vi "Final V1.vi"() -> ()   [LabVIEW 2021]
uses:
  <vilib>/MakerHub/LINX/Public/Sensors/Accelerometer/MPU60X0/AccelFullScaleRanges.ctl
  <vilib>/MakerHub/LINX/Public/Sensors/Accelerometer/MPU60X0/Clock Source.ctl
  <vilib>/MakerHub/LINX/Public/Sensors/Accelerometer/MPU60X0/DeviceAddresses.ctl
  <vilib>/MakerHub/LINX/Public/Sensors/Accelerometer/MPU60X0/GyroFullScaleRanges.ctl
  <vilib>/MakerHub/LINX/Public/Utilities/Open Serial.vi
  <vilib>/MakerHub/LINX/Public/Sensors/Motion/Servo/Servo Open One Channel.vi
  <vilib>/MakerHub/LINX/Public/Sensors/Motion/Servo/Servo Set Pulse Width One Channel.vi
  <vilib>/MakerHub/LINX/Public/Sensors/Motion/Servo/Servo Close One Channel.vi
  <vilib>/MakerHub/LINX/Public/Sensors/Motion/Servo/Servo.lvlib
  <vilib>/MakerHub/LINX/LMH-LINX.lvlib
  <vilib>/MakerHub/LINX/Public/Sensors/Accelerometer/MPU60X0/MPU60X0.lvlib
  <vilib>/Analysis/NI_AALPro.lvlib
panel:
  out "z position":dbl[](graph)
  out "y position":dbl[](graph)
  out "x position":dbl[](graph)
  out "acceleration graph":T1(graph)
  out "Acceleration Data (g)":T1
  in  "Servo 2":dbl(knob) scale=500.0..2400.0
  in  "Servo 1":dbl(knob) scale=500.0..2400.0
  in  "Stop Button":bool
  in  "Reset":bool
  in  "Serial Port":refnum<visa-resource-name>
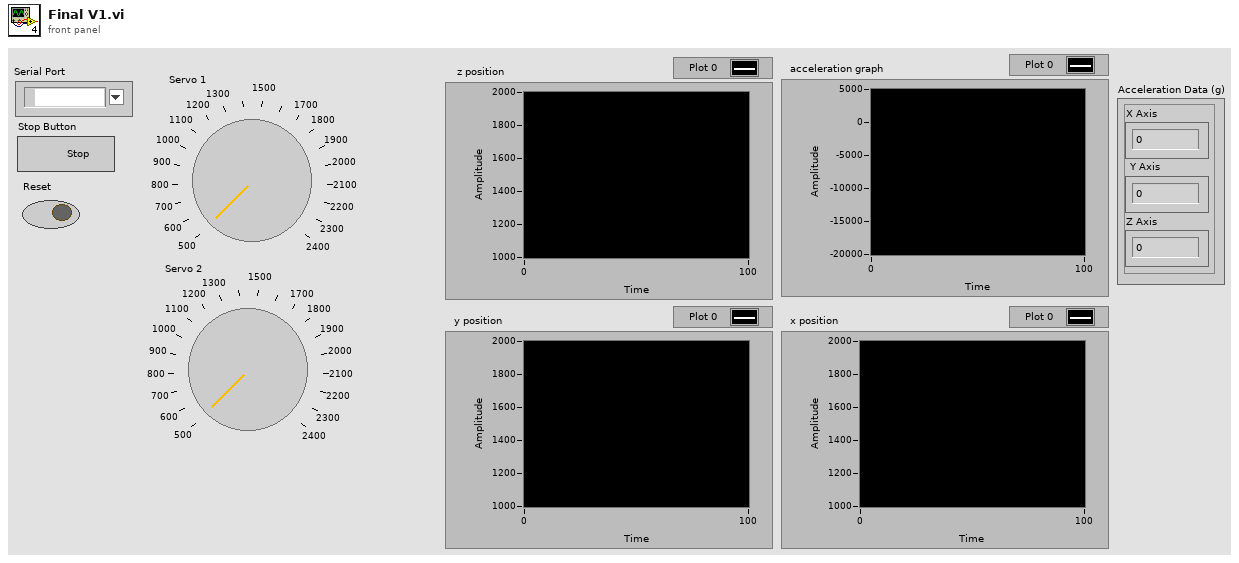
[diagram p1: front panel]
types:
  T1 = cluster{"X Axis":i16, "Y Axis":i16, "Z Axis":i16}
  T2 = typedef "LMH-LINX.lvlib/MPU60X0.lvlib/DeviceAddresses.ctl" = enum16{"0x68", "0x69"}
  T3 = typedef "LMH-LINX.lvlib/MPU60X0.lvlib/Clock Source.ctl" = enum8{"Internal 8MHz Osc", "PLL with X Gyro Ref", "PLL with Y Gyro Ref", "PLL with Z Gyro Ref", "PLL with ext 32.768 KHz Ref", "PLL with ext 19.2 MHz Ref", "Reserved", "Hold in reset"}
  T4 = typedef "LMH-LINX.lvlib/MPU60X0.lvlib/AccelFullScaleRanges.ctl" = enum16{"±2g", "±4g", "±8g", "±16g"}
  T5 = typedef "LMH-LINX.lvlib/MPU60X0.lvlib/GyroFullScaleRanges.ctl" = enum8{"±250 °/s", "±500 °/s", "±1000 °/s", "±2000 °/s"}
  T6 = typedef "LMH-LINX.lvlib/LINX Ref.ctl" = cluster{"IO":T7, "Interface":T8, "LINX Device Config":T9}
  T7 = typedef "LMH-LINX.lvlib/Platform.ctl" = enum16{"Remote", "Local"}
  T8 = typedef "LMH-LINX.lvlib/Interface.ctl" = enum16{"Serial", "TCP"}
  T9 = typedef "LMH-LINX.lvlib/Device.lvlib/LINX Device Config.ctl" = cluster{"Interface":T8, "COM Port":refnum<visa-resource-name>, "TCP Configuration":T10, "Device Family":u8, "Device ID":u8, "Device Name":string, "TCP Ref":refnum<k5>, "Channels":T11}
  T10 = typedef "LMH-LINX.lvlib/Device.lvlib/TCP Config.ctl" = cluster{"IP Address":string, "Port":u16}
  T11 = typedef "LMH-LINX.lvlib/Channels.ctl" = cluster{"DI":u8[], "DO":u8[], "AI":u8[], "AO":u8[], "PWM":u8[], "QE":u8[], "UART":u8[], "I2C 2":u8[], "SPI":u8[], "CAN":u8[], "Servo":u8[], "AI Ref (V)":dbl, "AI Resolution (Bits)":u8, "AO Ref (V)":dbl, "AO Resolution (Bits)":u8}
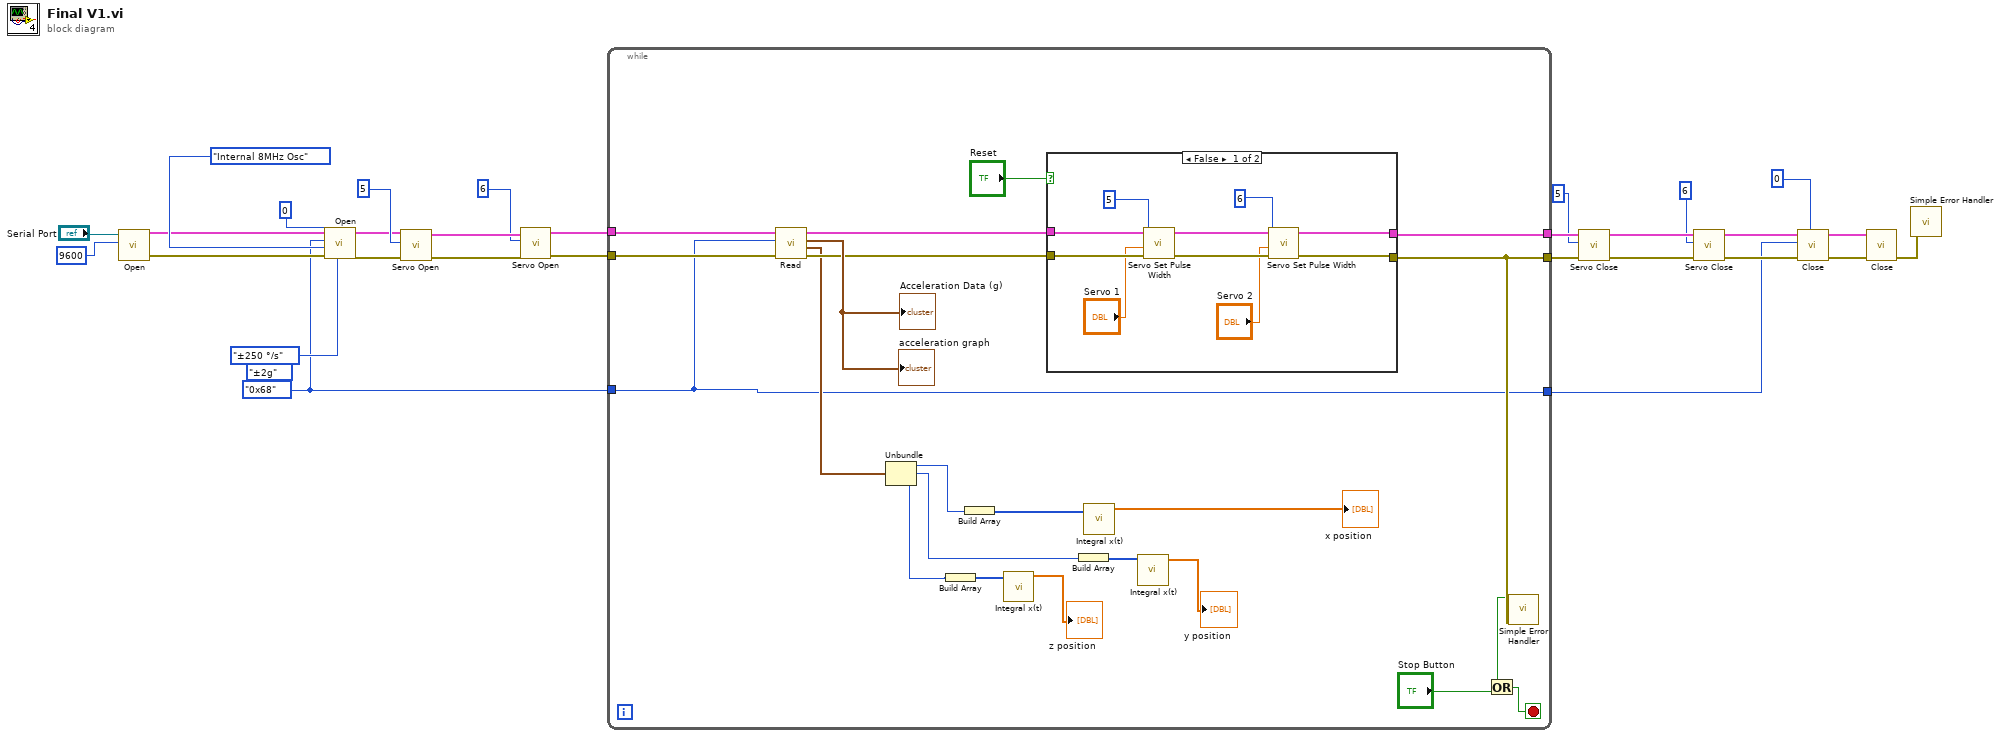
[diagram p0: block diagram]
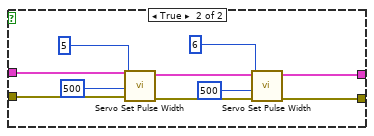
[diagram p2: hidden frame]
diagram:
  w7 = DeviceAddresses."0x68" ("I2C Slave Address")
  (unwired) GyroFullScaleRanges."±250 °/s" ("Gyro Full Scale Range")
  n1 = call-poly <vilib>:"Open.vi"("Baud Rate Override"=u32 9600, "Serial Port"="Serial Port") -> ("Error Out"=w8:errorcluster, "LINX Resource"=w11:T6)  [unwired: 7 in, 1 out]
  n2 = call <vilib>:"Open.vi"("Accel Full Scale Range"=AccelFullScaleRanges."±2g", "I2C Channel"=u8 0, "Error In"=w8, "Clock Source"=Clock_Source."Internal 8MHz Osc", "I2C Slave Address"=w7, "LINX Resource"=w11) -> ("Error Out"=w9:errorcluster, "LINX Resource"=w10:T6)  [unwired: 4 in]
  n3 = call-poly <vilib>:"Servo Open.vi"("Error In"=w9, "Servo Channel"=u8 5, "LINX Resource"=w10) -> ("Error Out"=w23:errorcluster, "LINX Resource"=w27:T6)  [unwired: 7 in]
  n4 = call-poly <vilib>:"Servo Open.vi"("Error In"=w23, "Servo Channel"=u8 6, "LINX Resource"=w27) -> ("Error Out"=w22:errorcluster, "LINX Resource"=w26:T6)  [unwired: 7 in]
  n5 = while {
    tunnel: w26 -> [w44]
    tunnel: [w50] -> w25
    tunnel: w22 -> [w42]
    tunnel: [w49] -> w21
    tunnel: w7 -> [w30]
    tunnel: [w30] -> w1
    stop <- w48 stop-if-true
    n6 = call <vilib>:"Read.vi"("Error In"=w42, "I2C Slave Address"=w30, "LINX Resource"=w44) -> ("Error Out"=w41:errorcluster, "Gyro  Data (dps)"=w34:T1, "Acceleration Data (g)"=→"Acceleration Data (g)" →"acceleration graph":T1, "LINX Resource"=w43:T6)  [unwired: 4 in, 1 out]
    n7 = Unbundle(w34) -> ("X Axis"=w40:i16, "Y Axis"=w33:i16, "Z Axis"=w35:i16)
    n8 = Build Array(w35) -> (w36:i16[])
    n9 = Build Array(w40) -> (w32:i16[])
    n10 = call <vilib>:"Integral x(t).vi"("X"=w36) -> ("Integral X"=→"z position":dbl[])  [unwired: 9 in, 1 out]
    n11 = case shown="False" "Reset" {
      tunnel: w43 -> [w59 w71]
      tunnel: [w58 w69] -> w50
      tunnel: w41 -> [w57 w68]
      tunnel: [w56 w66] -> w49
      frame False {
        n12 = call-poly <vilib>:"Servo Set Pulse Width.vi"("Error In"=w57, "Pulse Width (uS)"="Servo 1", "Servo Channel"=u8 5, "LINX Resource"=w59) -> ("Error Out"=w60:errorcluster, "LINX Resource"=w61:T6)  [unwired: 6 in]
        n13 = call-poly <vilib>:"Servo Set Pulse Width.vi"("Error In"=w60, "Pulse Width (uS)"="Servo 2", "Servo Channel"=u8 6, "LINX Resource"=w61) -> ("Error Out"=w56:errorcluster, "LINX Resource"=w58:T6)  [unwired: 6 in]
      }
      frame True {
        n14 = call-poly <vilib>:"Servo Set Pulse Width.vi"("Error In"=w68, "Pulse Width (uS)"=u16 500, "Servo Channel"=u8 5, "LINX Resource"=w71) -> ("Error Out"=w67:errorcluster, "LINX Resource"=w70:T6)  [unwired: 6 in]
        n15 = call-poly <vilib>:"Servo Set Pulse Width.vi"("Error In"=w67, "Pulse Width (uS)"=u16 500, "Servo Channel"=u8 6, "LINX Resource"=w70) -> ("Error Out"=w66:errorcluster, "LINX Resource"=w69:T6)  [unwired: 6 in]
      }
    }
    n16 = Build Array(w33) -> (w38:i16[])
    n17 = call <vilib>:"Integral x(t).vi"("X"=w32) -> ("Integral X"=→"x position":dbl[])  [unwired: 9 in, 1 out]
    n18 = call <vilib>:"Integral x(t).vi"("X"=w38) -> ("Integral X"=→"y position":dbl[])  [unwired: 9 in, 1 out]
    n19 = call <vilib>:"Simple Error Handler.vi"("error in (no error)"=w49) -> ("error?"=w47:bool)  [unwired: 4 in, 4 out]
    n20 = Or(x=w47, y="Stop Button") -> (x .or. y?=w48:bool)
  }
  n21 = call-poly <vilib>:"Servo Close.vi"("Error In"=w21, "Servo Channel"=u8 5, "LINX Resource"=w25) -> ("Error Out"=w20:errorcluster, "LINX Resource"=w24:T6)  [unwired: 7 in]
  n22 = call-poly <vilib>:"Servo Close.vi"("Error In"=w20, "Servo Channel"=u8 6, "LINX Resource"=w24) -> ("Error Out"=w3:errorcluster, "LINX Resource"=w5:T6)  [unwired: 7 in]
  n23 = call <vilib>:"Close.vi"("I2C Channel (0)"=u8 0, "Error In"=w3, "I2C Slave Address (0)"=w1, "LINX Resource"=w5) -> ("Error Out"=w2:errorcluster, "LINX Resource"=w4:T6)  [unwired: 6 in]
  n24 = call <vilib>:"Close.vi"("Error In"=w2, "LINX Resource"=w4) -> ("Error Out"=w28:errorcluster)  [unwired: 9 in]
  n25 = call <vilib>:"Simple Error Handler.vi"("error in (no error)"=w28) -> ()  [unwired: 4 in, 5 out]
